vi "Create All Message Queues.vi"(8 "Error In":errorcluster) -> (0 "Error Out":errorcluster, 3 "Message Queues out":T1)   [LabVIEW 2017]
doc: "This VI creates and initializes all the message queues for your application. If your application requires more than one message queue, right-click the \"Message Queues\" constant above and select Open Type Def. Add the new Message Queue(s) to the type definition, then initialize them in this VI."
uses:
  Typedefs/All Message Queues.ctl
  Typedefs/Message Cluster.ctl
  Typedefs/Logging queue element.ctl
  Typedefs/Imaging Protocols enum.ctl
  Typedefs/Frame Size.ctl
  Typedefs/Acquired points count.ctl
  Global Variables/gl_Queues.vi
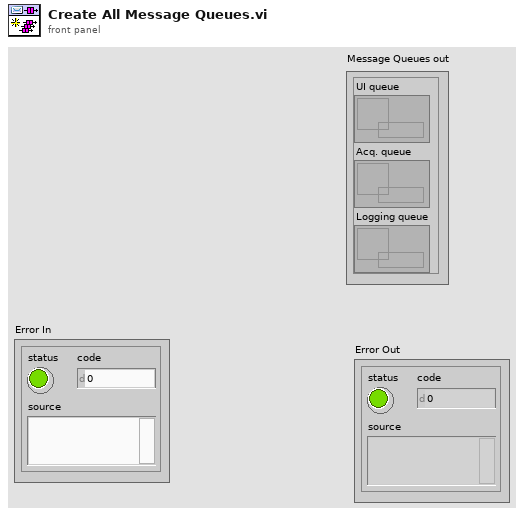
[diagram p1: front panel]
types:
  T1 = typedef "All Message Queues.ctl" = cluster{"UI queue":refnum<queue>, "Acq. queue":refnum<queue>, "Logging queue":refnum<queue>}
  T2 = typedef "Logging queue element.ctl" = cluster{"Imaging Protocol":T3, "Number of Trials":u16, "Frame Size":T4, "# Averaged frames":u16, "Dwell time (us)":dbl, "Index of Z-plane":i32, "Timelapse?":bool, "Logging process is active":bool, "Speed logging enabled":bool, "tdms file ref":refnum<k34>, "path":path, "Trial Number":i32, "Expected # points acquired":bool, "Manually stopped":bool, "Ch0 data":u32[], "Ch1 data":u32[], "Ref Data":u32[], "Last trial":bool, "Ref Dwell time (us)":dbl, "# Ref Averaged frames":u16, "Ref X Length":u16, "Ref Y Length":u16, "Points acquired":T5}
  T3 = typedef "Imaging Protocols enum.ctl" = enum16{"AOL Z-Stack", "Motor Z Stack", "Functional Acquisition", "Single Plane Acquisition", "Volume Acquisition", "Live Imaging", "Live Plane Imaging", "Live Volume Imaging"}
  T4 = typedef "Frame Size.ctl" = u16
  T5 = typedef "Acquired points count.ctl" = cluster{"Ch0 last trial":u64, "Ch1 last trial":u64, "All trials":u64}
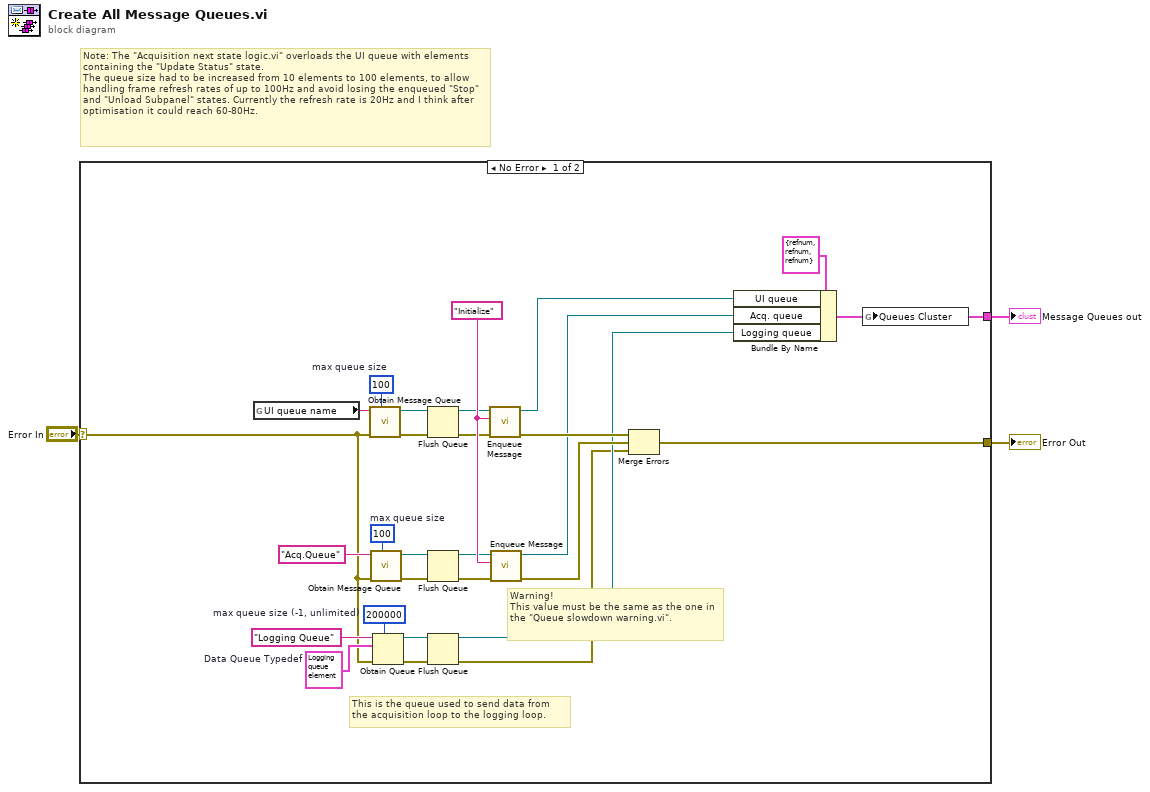
[diagram p0: block diagram]
diagram:
  # "Note: The \"Acquisition next state logic.vi\" overloads the UI queue with elements containing the \"Update Status\" state.\nThe queue size had to be increased from 10 elements to 100 elements, to allow handling frame refresh rates of up to 100Hz and avoid losing the enqueued \"Stop\" and \"Unload Subpanel\" states. Currently the refresh rate is 20Hz and I think after optimisation it could reach 60-80Hz."
  n1 = case shown="No Error" "Error In" {
    selector: "Error In" -> [w8 w32]
    tunnel: [w27 w32] -> w2
    tunnel: [w5 _] -> w3
    frame No Error {
      w6 = 100  # max queue size
      w7 = 100  # max queue size
      w15 = T2 {"Imaging Protocol"=enum."AOL Z-Stack", "Number of Trials"=0, "Frame Size"=0, "# Averaged frames"=0, "Dwell time (us)"=0.0, "Index of Z-plane"=0, "Timelapse?"=FALSE, "Logging process is active"=FALSE, "Speed logging enabled"=FALSE, "tdms file ref"=refnum, "path"=path "", "Trial Number"=0, "Expected # points acquired"=FALSE, "Manually stopped"=FALSE, "Ch0 data"=[], "Ch1 data"=[], "Ref Data"=[], "Last trial"=FALSE, "Ref Dwell time (us)"=0.0, "# Ref Averaged frames"=0, "Ref X Length"=0, "Ref Y Length"=0, "Points acquired"={"Ch0 last trial"=0, "Ch1 last trial"=0, "All trials"=0}}  # Data Queue Typedef
      w13 = 200000  # max queue size (-1, unlimited)
      w30 = "Initialize" ("Message")
      # "Warning!\nThis value must be the same as the one in the \"Queue slowdown warning.vi\"."
      # "This is the queue used to send data from \nthe acquisition loop to the logging loop."
      n2 = global read "gl_Queues.vi" "UI queue name"() -> (w4:string)
      n3 = call "Obtain Message Queue.vi"("max queue size (-1, unlimited)"=w6, "error in (no error)"=w8, "Queue name"=w4) -> ("error out"=w22:errorcluster, "Message Queue"=w24:refnum<queue>)  [unwired: 7 in]
      n4 = call "Obtain Message Queue.vi"("max queue size (-1, unlimited)"=w7, "error in (no error)"=w8, "Queue name"="Acq.Queue") -> ("error out"=w19:errorcluster, "Message Queue"=w20:refnum<queue>)  [unwired: 7 in]
      n5 = Obtain Queue(max queue size (-1, unlimited)=w13, name (unnamed)="Logging Queue", element data type=w15, error in (no error)=w8) -> (queue out=w12:refnum<queue>, error out=w9:errorcluster)  [unwired: 1 in, 1 out]
      n6 = Flush Queue(queue=w24, error in (no error)=w22) -> (queue out=w23:refnum<queue>, error out=w21:errorcluster)  [unwired: 1 out]
      n7 = Flush Queue(queue=w20, error in (no error)=w19) -> (queue out=w17:refnum<queue>, error out=w18:errorcluster)  [unwired: 1 out]
      n8 = Flush Queue(queue=w12, error in (no error)=w9) -> (queue out=w11:refnum<queue>, error out=w10:errorcluster)  [unwired: 1 out]
      n9 = call "Enqueue Message.vi"("error in (no error)"=w21, "Message"=w30, "Queue"=w23) -> ("error out"=w31:errorcluster, "Queue out"=w29:refnum<queue>)  [unwired: 7 in]
      n10 = call "Enqueue Message.vi"("error in (no error)"=w18, "Message"=w30, "Queue"=w17) -> ("error out"=w26:errorcluster, "Queue out"=w28:refnum<queue>)  [unwired: 7 in]
      n11 = Merge Errors(w31, w26, w10) -> (w27:errorcluster)
      n12 = Bundle By Name(cluster=T1 {"UI queue"=refnum, "Acq. queue"=refnum, "Logging queue"=refnum} ("Message Queues"), "UI queue"=w29, "Acq. queue"=w28, "Logging queue"=w11) -> (w5:T1)
      n13 = global write "gl_Queues.vi" "Queues Cluster"(w5) -> ()
    }
    frame Error {
    }
  }
  "Message Queues out" <- w3
  "Error Out" <- w2
